vi "Rolling Display.vi"(6 "Input Data":dbl[][](array[numeric]), 8 "Channels in Use":T2, 9 "Old Data":dbl[][](array[numeric]), 10 "Sample Rate":i32, 11 "Display Size":T3(ring)) -> (1 "Output Array Values":dbl[][](array[numeric]), 3 "Output Waveform Cluster":T1)   [LabVIEW 2014]
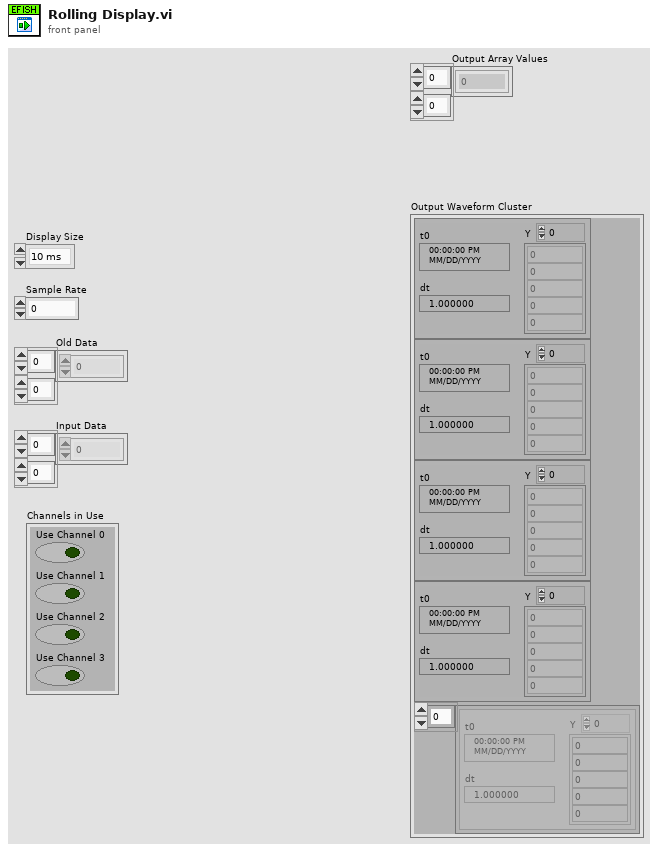
[diagram p1: front panel]
types:
  T1 = cluster{"Waveform":waveform(dbl), "Waveform":waveform(dbl), "Waveform":waveform(dbl), "Waveform":waveform(dbl), waveform(dbl)[]}
  T2 = cluster{"Use Channel 0":bool, "Use Channel 1":bool, "Use Channel 2":bool, "Use Channel 3":bool}
  T3 = enum16{"10 ms", "100 ms", "1 Second", "10 sec", "30 sec"}
  T4 = cluster{waveform(dbl), waveform(dbl), waveform(dbl), waveform(dbl), waveform(dbl)[]}
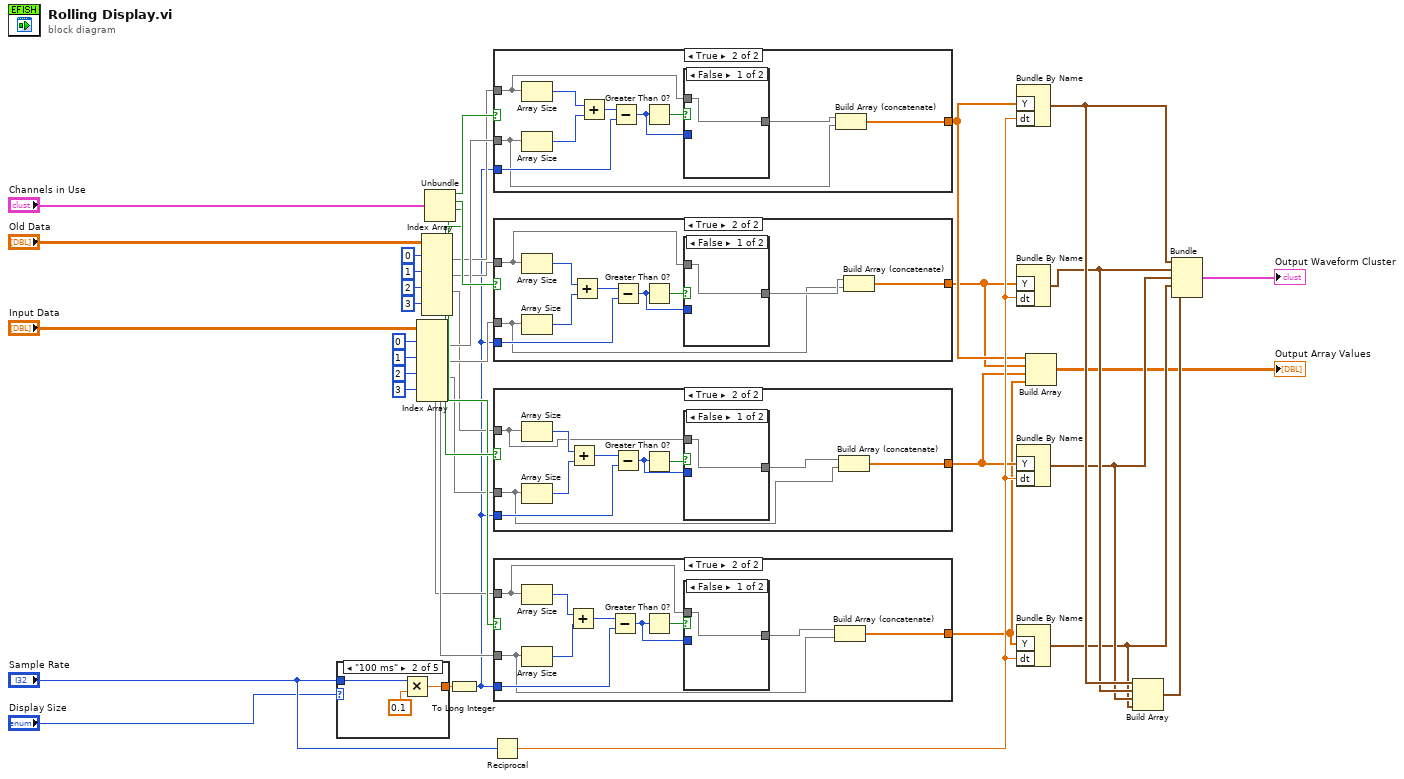
[diagram p0: block diagram]
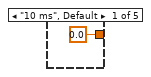
[diagram p2: hidden frame]
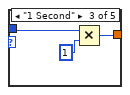
[diagram p3: hidden frame]
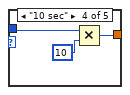
[diagram p4: hidden frame]
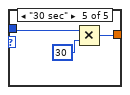
[diagram p5: hidden frame]
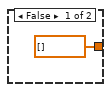
[diagram p6: hidden frame]
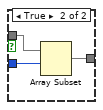
[diagram p7: hidden frame]
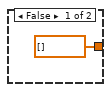
[diagram p8: hidden frame]
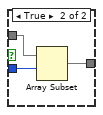
[diagram p9: hidden frame]
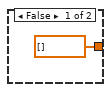
[diagram p10: hidden frame]
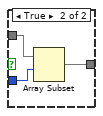
[diagram p11: hidden frame]
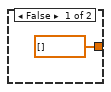
[diagram p12: hidden frame]
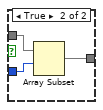
[diagram p13: hidden frame]
diagram:
  n1 = case shown="\"100 ms\"" "Display Size" {
    tunnel: "Sample Rate" -> [_ w43 w45 w48 w51]
    tunnel: [0.0 w41 w46 w49 w52] -> w17
    frame "10 ms", Default {
    }
    frame "100 ms" {
      n2 = Multiply(x=w43, y=0.1) -> (x*y=w41:dbl)
    }
    frame "1 Second" {
      n3 = Multiply(x=w45, y=1) -> (x*y=w46:i32)
    }
    frame "10 sec" {
      n4 = Multiply(x=w48, y=10) -> (x*y=w49:i32)
    }
    frame "30 sec" {
      n5 = Multiply(x=w51, y=30) -> (x*y=w52:i32)
    }
  }
  n6 = Index Array(array="Input Data", index (row) #1=0 ("index (row)"), index (row) #2=1 ("index (row)"), index (row) #3=2 ("index (row)"), index (row) #4=3 ("index (row)")) -> (element #1=w26:dbl[], element #2=w25:dbl[], element #3=w24:dbl[], element #4=w23:dbl[])  [unwired: 4 in]
  n7 = Index Array(array="Old Data", index (row) #1=0 ("index (row)"), index (row) #2=1 ("index (row)"), index (row) #3=2 ("index (row)"), index (row) #4=3 ("index (row)")) -> (element #1=w21:dbl[], element #2=w20:dbl[], element #3=w19:dbl[], element #4=w18:dbl[])  [unwired: 4 in]
  n8 = Unbundle("Channels in Use") -> ("Use Channel 0"=w34:bool, "Use Channel 1"=w33:bool, "Use Channel 2"=w32:bool, "Use Channel 3"=w31:bool)
  n9 = To Long Integer(number=w17) -> (32bit integer=w16:i32)
  n10 = Reciprocal(x="Sample Rate") -> (1/x=w15:dbl)
  n11 = case shown="True" w34 {
    tunnel: w26 -> [_ w54]
    tunnel: w21 -> [_ w57]
    tunnel: w16 -> [_ w60]
    tunnel: [dbl[] [] w56] -> w9
    frame False {
    }
    frame True {
      n12 = Array Size(array=w57) -> (size(s)=w63:i32)
      n13 = Array Size(array=w54) -> (size(s)=w62:i32)
      n14 = Add(x=w63, y=w62) -> (x+y=w61:i32)
      n15 = Subtract(x=w61, y=w60) -> (x-y=w58:i32)
      n16 = Greater Than 0?(x=w58) -> (x > 0?=w59:bool)
      n17 = case shown="False" w59 {
        tunnel: w58 -> [_ w67]
        tunnel: w57 -> [w64 w66]
        tunnel: [w64 w65] -> w55
        frame False {
        }
        frame True {
          n18 = Array Subset(array=w66, index=w67) -> (w65:dbl[])  [unwired: 1 in]
        }
      }
      n19 = Build Array (concatenate)(w55, w54) -> (w56:dbl[])
    }
  }
  n20 = case shown="True" w33 {
    tunnel: w25 -> [_ w69]
    tunnel: w20 -> [_ w72]
    tunnel: w16 -> [_ w75]
    tunnel: [dbl[] [] w71] -> w8
    frame False {
    }
    frame True {
      n21 = Array Size(array=w72) -> (size(s)=w78:i32)
      n22 = Array Size(array=w69) -> (size(s)=w77:i32)
      n23 = Add(x=w78, y=w77) -> (x+y=w76:i32)
      n24 = Subtract(x=w76, y=w75) -> (x-y=w73:i32)
      n25 = Greater Than 0?(x=w73) -> (x > 0?=w74:bool)
      n26 = case shown="False" w74 {
        tunnel: w73 -> [_ w82]
        tunnel: w72 -> [w79 w81]
        tunnel: [w79 w80] -> w70
        frame False {
        }
        frame True {
          n27 = Array Subset(array=w81, index=w82) -> (w80:dbl[])  [unwired: 1 in]
        }
      }
      n28 = Build Array (concatenate)(w70, w69) -> (w71:dbl[])
    }
  }
  n29 = case shown="True" w32 {
    tunnel: w24 -> [_ w84]
    tunnel: w19 -> [_ w87]
    tunnel: w16 -> [_ w90]
    tunnel: [dbl[] [] w86] -> w7
    frame False {
    }
    frame True {
      n30 = Array Size(array=w87) -> (size(s)=w93:i32)
      n31 = Array Size(array=w84) -> (size(s)=w92:i32)
      n32 = Add(x=w93, y=w92) -> (x+y=w91:i32)
      n33 = Subtract(x=w91, y=w90) -> (x-y=w88:i32)
      n34 = Greater Than 0?(x=w88) -> (x > 0?=w89:bool)
      n35 = case shown="False" w89 {
        tunnel: w88 -> [_ w97]
        tunnel: w87 -> [w94 w96]
        tunnel: [w94 w95] -> w85
        frame False {
        }
        frame True {
          n36 = Array Subset(array=w96, index=w97) -> (w95:dbl[])  [unwired: 1 in]
        }
      }
      n37 = Build Array (concatenate)(w85, w84) -> (w86:dbl[])
    }
  }
  n38 = case shown="True" w31 {
    tunnel: w23 -> [_ w100]
    tunnel: w18 -> [_ w102]
    tunnel: w16 -> [_ w105]
    tunnel: [dbl[] [] w101] -> w6
    frame False {
    }
    frame True {
      n39 = Array Size(array=w102) -> (size(s)=w108:i32)
      n40 = Array Size(array=w100) -> (size(s)=w107:i32)
      n41 = Add(x=w108, y=w107) -> (x+y=w106:i32)
      n42 = Subtract(x=w106, y=w105) -> (x-y=w103:i32)
      n43 = Greater Than 0?(x=w103) -> (x > 0?=w104:bool)
      n44 = case shown="False" w104 {
        tunnel: w103 -> [_ w112]
        tunnel: w102 -> [w109 w111]
        tunnel: [w109 w110] -> w99
        frame False {
        }
        frame True {
          n45 = Array Subset(array=w111, index=w112) -> (w110:dbl[])  [unwired: 1 in]
        }
      }
      n46 = Build Array (concatenate)(w99, w100) -> (w101:dbl[])
    }
  }
  n47 = Bundle By Name("Y"=w9, "dt"=w15) -> (w14:waveform(dbl))  [unwired: 1 in]
  n48 = Bundle By Name("Y"=w8, "dt"=w15) -> (w13:waveform(dbl))  [unwired: 1 in]
  n49 = Bundle By Name("Y"=w7, "dt"=w15) -> (w12:waveform(dbl))  [unwired: 1 in]
  n50 = Bundle By Name("Y"=w6, "dt"=w15) -> (w11:waveform(dbl))  [unwired: 1 in]
  n51 = Build Array(w9, w8, w7, w6) -> (→"Output Array Values":dbl[][])
  n52 = Build Array(w14, w13, w12, w11) -> (w10:waveform(dbl)[])
  n53 = Bundle(w14, w13, w12, w11, w10) -> (→"Output Waveform Cluster":T4)  [unwired: 1 in]
